vi "Dispose.vi"(8 "error in (no error)":errorcluster, 11 "ByRef":refnum<class "MazeGame.lvclass">) -> (0 "error out":errorcluster)   [LabVIEW 2020, in "FactoryMethod.lvlib" / "MazeGame.lvclass"]
uses:
  MazeGame.lvclass
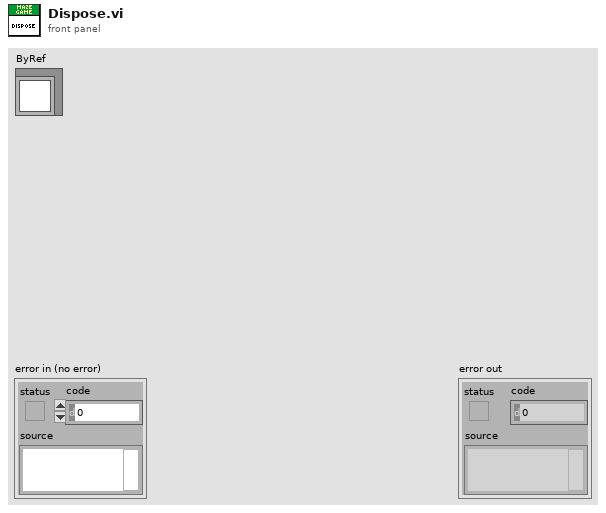
[diagram p1: front panel]
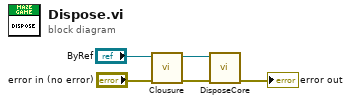
[diagram p0: block diagram]
diagram:
  n1 = call-dynamic "Clousure.vi"("error in (no error)"="error in (no error)", "MazeGame"="ByRef") -> ("error out"=w1:errorcluster, "MazeGame"=w2:refnum<class "MazeGame.lvclass">)  [unwired: 8 in]
  n2 = call-dynamic "DisposeCore.vi"("error in (no error)"=w1, "MazeGame"=w2) -> ("error out"=→"error out":errorcluster)  [unwired: 8 in, 1 out]
